vi "Write Files.vi"(8 "error in (no error)":errorcluster, 11 "CHM Generator in":refnum<class "CHM Generator.lvclass">) -> (0 "error out":errorcluster, 3 "CHM Generator out":refnum<class "CHM Generator.lvclass">)   [LabVIEW 2015, in "CHM Generator.lvclass"]
uses:
  CHM Generator.lvclass
  CHM Generator.lvclass/CHM Generator.ctl
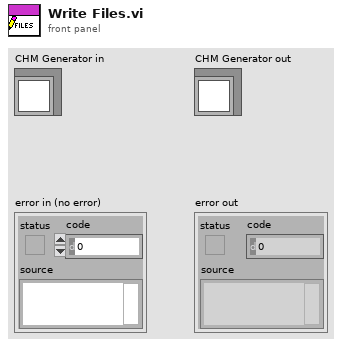
[diagram p1: front panel]
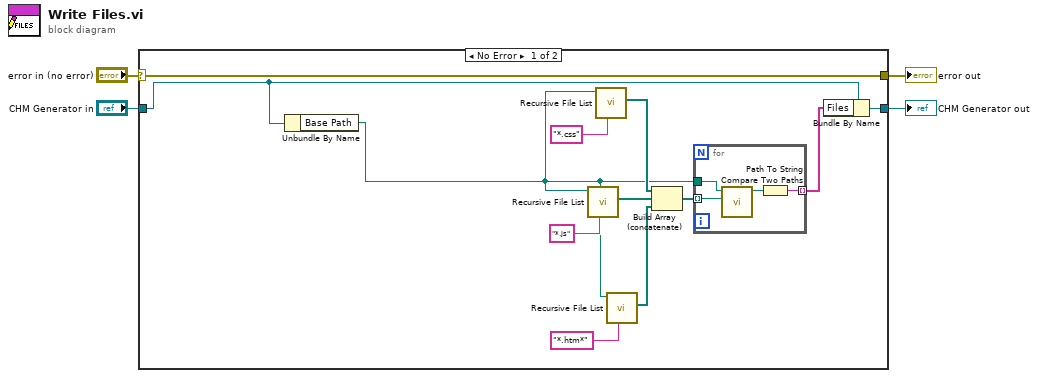
[diagram p0: block diagram]
diagram:
  n1 = case shown="No Error" "error in (no error)" {
    selector: "error in (no error)" -> [w16 w21]
    tunnel: [w16 w21] -> w3
    tunnel: [w15 w22] -> w1
    tunnel: "CHM Generator in" -> [w6 w22]
    frame No Error {
      n2 = Unbundle By Name(w6) -> ("Base Path"=w5:path)
      n3 = call <vilib>:"Recursive File List.vi"("pattern"="*.js", "Folder Path"=w5) -> ("All Files in Dir"=w11:path[])  [unwired: 5 in, 4 out]
      n4 = call <vilib>:"Recursive File List.vi"("pattern"="*.css", "Folder Path"=w5) -> ("All Files in Dir"=w9:path[])  [unwired: 5 in, 4 out]
      n5 = call <vilib>:"Recursive File List.vi"("pattern"="*.htm*", "Folder Path"=w5) -> ("All Files in Dir"=w12:path[])  [unwired: 5 in, 4 out]
      n6 = Build Array (concatenate)(w9, w11, w12) -> (w8:path[])
      n7 = for {
        tunnel: w5 -> [w20]
        tunnel: w8 -> [w19] mode=indexing
        tunnel: [w17] -> w7 mode=indexing
        n8 = call <vilib>:"Compare Two Paths.vi"("Path 2"=w19, "Path 1"=w20) -> ("Relative Path from 1 to 2"=w18:path)  [unwired: 6 in, 3 out]
        n9 = Path To String(path=w18) -> (string=w17:string)
      }
      n10 = Bundle By Name(cluster=w6, "Files"=w7) -> (w15:refnum<class "CHM Generator.lvclass">)
    }
    frame Error {
    }
  }
  "error out" <- w3
  "CHM Generator out" <- w1
